vi "Read Key (I32).vi"(7 "section":string, 8 "error in (no error)":errorcluster, 9 "default value":i32, 10 "key":string, 11 "refnum":T1) -> (0 "error out":errorcluster, 1 "value":i32, 2 "found?":bool, 3 "refnum out":T1)   [LabVIEW 2009]
doc: "Reads a value associated with a key in a specified section from the configuration data identified by <B>refnum</B>. If the key does not exist, the VI returns the default value. You can use this polymorphic VI to read the following types of values from a key: Boolean, double-precision numeric, signed integer, path, string, and unsigned integer. The data type you wire to the <B>default value</B> input determines the polymorphic instance to use."
uses:
  <vilib>/Utility/config.llb/Config Data RefNum.ctl
  <vilib>/Utility/config.llb/NI_LVConfig.lvlib
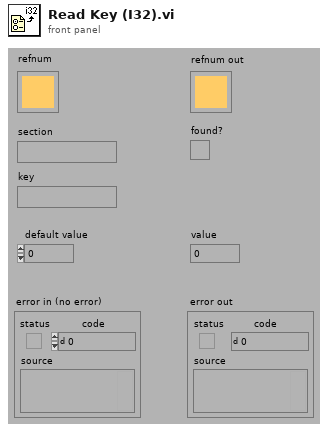
[diagram p1: front panel]
types:
  T1 = typedef "NI_LVConfig.lvlib/Config Data RefNum.ctl" = refnum<k1>
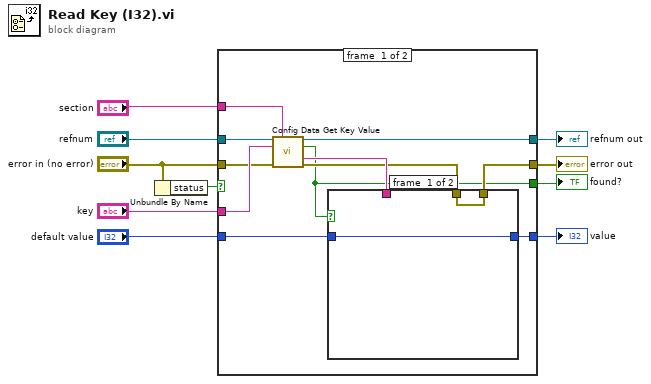
[diagram p0: block diagram]
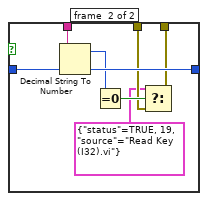
[diagram p2: hidden frame]
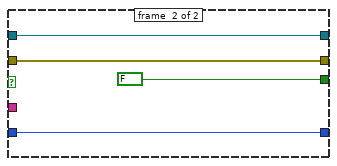
[diagram p3: hidden frame]
diagram:
  n1 = Unbundle By Name("error in (no error)") -> ("status"=w10:bool)
  n2 = case shown="False" w10 {
    tunnel: [w18 w34] -> w9
    tunnel: [w12 w35] -> w8
    tunnel: "refnum" -> [w14 w34]
    tunnel: "error in (no error)" -> [w15 w35]
    tunnel: "section" -> [w21 _]
    tunnel: "key" -> [w20 _]
    tunnel: [w11 FALSE ("section exists?")] -> w7
    tunnel: [w19 w33] -> w6
    tunnel: "default value" -> [w16 w33]
    frame #0 {
      n3 = call "Config Data Get Key Value.vi"("config data"=w14, "section"=w21, "key"=w20, "error in (no error)"=w15) -> ("config data out"=w18:T1, "key exists?"=w11:bool, "key value"=w17:string, "error out"=w13:errorcluster)  [unwired: 6 in, 2 out]
      n4 = case shown="True" w11 {
        tunnel: [w23 w31] -> w19
        tunnel: w17 -> [_ w30]
        tunnel: w16 -> [w23 w29]
        tunnel: w13 -> [w22 w26]
        tunnel: [w22 w24] -> w12
        frame #0 {
        }
        frame #1 {
          n5 = Decimal String To Number(string=w30, default (0L)=w29) -> (offset past number=w28:i32, number=w31:i32)  [unwired: 1 in]
          n6 = Equal To 0?(x=w28) -> (x = 0?=w27:bool)
          n7 = Select(t=cluster{"status":bool, u16, "source":string} {"status"=TRUE, 19, "source"="Read Key (I32).vi"} ("f"), s=w27, f=w26) -> (s? t:f=w24:errorcluster)
        }
      }
    }
    frame #1 {
    }
  }
  "error out" <- w8
  "refnum out" <- w9
  "value" <- w6
  "found?" <- w7
